vi "Consume RPC Param Data.vi"(8 "Param Name":string, 9 "VI in":refnum<vi>, 10 "type":u8, 11 "RPC String in":string) -> (0 "Value String":string, 1 "Value":variant, 2 "string out":string, 3 "Issue":bool)   [LabVIEW 2017]
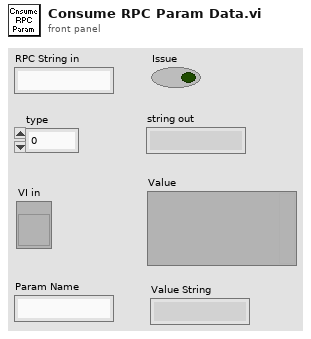
[diagram p1: front panel]
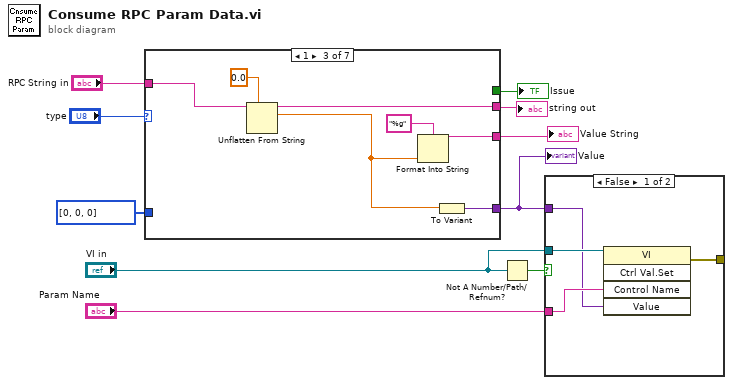
[diagram p0: block diagram]
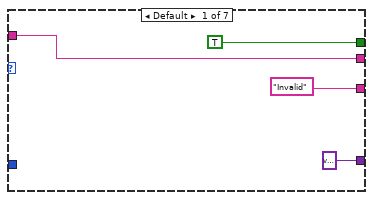
[diagram p3: hidden frame]
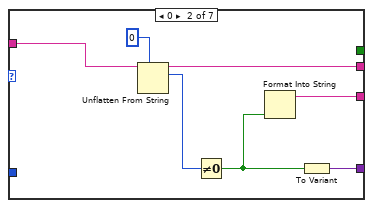
[diagram p4: hidden frame]
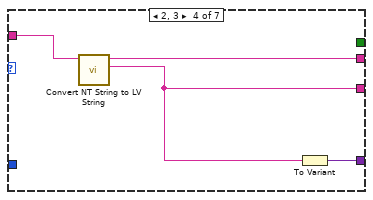
[diagram p5: hidden frame]
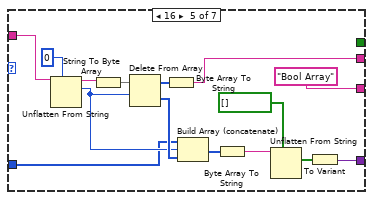
[diagram p6: hidden frame]
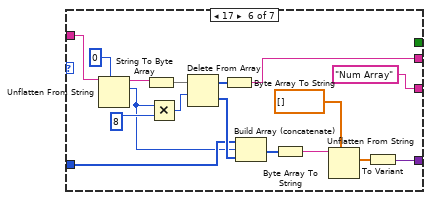
[diagram p7: hidden frame]
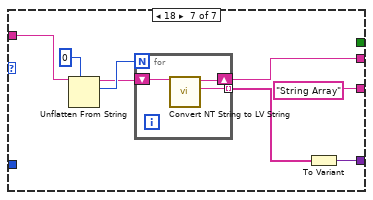
[diagram p8: hidden frame]
diagram:
  n1 = case shown="1" "type" {
    tunnel: [w13 w20 w27 w32 w43 w60 w69] -> w8
    tunnel: [TRUE _ _ _ _ _ _] -> w9
    tunnel: "RPC String in" -> [w13 w19 w26 w31 w42 w59 w68]
    tunnel: [variant ("Variant") w18 w25 w30 w35 w54 w67] -> w3
    tunnel: u8[] [0, 0, 0] -> [_ _ _ _ w39 w57 _]
    tunnel: ["Invalid" w15 w24 w29 "Bool Array" "Num Array" "String Array"] -> w1
    frame Default {
    }
    frame 0 {
      n2 = Unflatten From String(type=u8 0, binary string=w19) -> (rest of the binary string=w20:string, value=w17:u8)  [unwired: 3 in, 1 out]
      n3 = Not Equal To 0?(x=w17) -> (x != 0?=w16:bool)
      n4 = Format Into String(w16) -> (resulting string=w15:string)  [unwired: 3 in, 1 out]
      n5 = To Variant(anything=w16) -> (Variant=w18:variant)
    }
    frame 1 {
      n6 = Unflatten From String(type=0.0, binary string=w26) -> (rest of the binary string=w27:string, value=w23:dbl)  [unwired: 3 in, 1 out]
      n7 = Format Into String(format string="%g", w23) -> (resulting string=w24:string)  [unwired: 2 in, 1 out]
      n8 = To Variant(anything=w23) -> (Variant=w25:variant)
    }
    frame 2, 3 {
      n9 = call <vilib>:"Convert NT String to LV String.vi"("Buffer in"=w31) -> ("String Contents"=w29:string, "Remaining String"=w32:string)  [unwired: 8 in, 1 out]
      n10 = To Variant(anything=w29) -> (Variant=w30:variant)
    }
    frame 16 {
      n11 = Unflatten From String(type=u8 0 ("bytes to read"), binary string=w42) -> (rest of the binary string=w46:string, value=w40:u8)  [unwired: 3 in, 1 out]
      n12 = String To Byte Array(string=w46) -> (unsigned byte array=w45:u8[])
      n13 = Delete From Array(array=w45, length=w40) -> (deleted portion=w41:u8[], array with subset deleted=w44:u8[])  [unwired: 1 in]
      n14 = Byte Array To String(unsigned byte array=w44) -> (string=w43:string)
      n15 = Build Array (concatenate)(w39, w40, w41) -> (w38:u8[])
      n16 = Byte Array To String(unsigned byte array=w38) -> (string=w37:string)
      n17 = Unflatten From String(type=bool[] [], binary string=w37) -> (value=w34:bool[])  [unwired: 3 in, 2 out]
      n18 = To Variant(anything=w34) -> (Variant=w35:variant)
    }
    frame 17 {
      n19 = Unflatten From String(type=u8 0 ("bytes to read"), binary string=w59) -> (rest of the binary string=w63:string, value=w50:u8)  [unwired: 3 in, 1 out]
      n20 = String To Byte Array(string=w63) -> (unsigned byte array=w62:u8[])
      n21 = Multiply(x=w50, y=8) -> (x*y=w49:i32)
      n22 = Delete From Array(array=w62, length=w49) -> (deleted portion=w58:u8[], array with subset deleted=w61:u8[])  [unwired: 1 in]
      n23 = Byte Array To String(unsigned byte array=w61) -> (string=w60:string)
      n24 = Build Array (concatenate)(w57, w50, w58) -> (w56:u8[])
      n25 = Byte Array To String(unsigned byte array=w56) -> (string=w55:string)
      n26 = Unflatten From String(type=dbl[] [], binary string=w55) -> (value=w53:dbl[])  [unwired: 3 in, 2 out]
      n27 = To Variant(anything=w53) -> (Variant=w54:variant)
    }
    frame 18 {
      n28 = Unflatten From String(type=u8 0 ("bytes to read"), binary string=w68) -> (rest of the binary string=w70:string, value=w71:u8)  [unwired: 3 in, 1 out]
      n29 = for {
        N: w71 -> [_]
        shift-right: [w74] -> w69
        shift-left: w70 -> [w75]
        tunnel: [w73] -> w66 mode=indexing
        n30 = call <vilib>:"Convert NT String to LV String.vi"("Buffer in"=w75) -> ("String Contents"=w73:string, "Remaining String"=w74:string)  [unwired: 8 in, 1 out]
      }
      n31 = To Variant(anything=w66) -> (Variant=w67:variant)
    }
  }
  "Issue" <- w9
  "string out" <- w8
  "Value" <- w3
  "Value String" <- w1
  n32 = Not A Number/Path/Refnum?(number/path/refnum="VI in") -> (NaN/Path/Refnum?=w6:bool)
  n33 = case shown="False" w6 {
    tunnel: "Param Name" -> [w78 _]
    tunnel: "VI in" -> [w79 _]
    tunnel: w3 -> [w77 _]
    tunnel: [w76 _] -> _
    frame False {
      n34 = invoke class="VI" method="Ctrl Val.Set"(reference=w79, "Control Name"=w78, "Value"=w77) -> (error out=w76:errorcluster)  [unwired: 2 in, 4 out]
    }
    frame True {
    }
  }
